vi "Obtain ACQ Data Queue.vi"(8 "error in (no error)":errorcluster) -> (0 "error out":errorcluster, 3 "ACQ Data Queue out":refnum<queue>)   [LabVIEW 2014, in "WINFAS 2 Data Queue.lvlib"]
uses:
  WINFAS 2 Data Queue.lvlib
  Acquisition Data 1 Sample Cluster.ctl
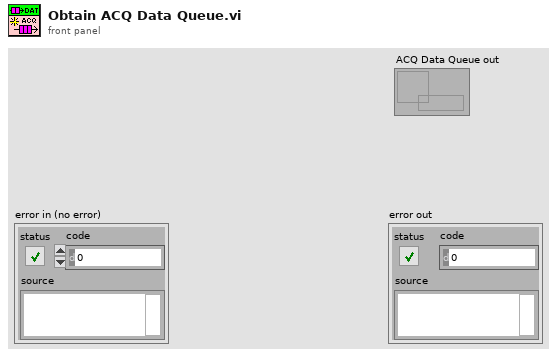
[diagram p1: front panel]
types:
  T1 = typedef "WINFAS 2 Data Queue.lvlib/Acquisition Data 1 Sample Cluster.ctl" = cluster{"TDX":sgl[], "Encoder":sgl}
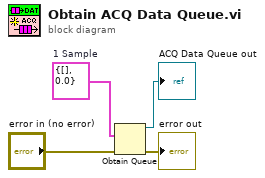
[diagram p0: block diagram]
diagram:
  w2 = T1 {"TDX"=[], "Encoder"=0.0}  # 1 Sample
  n1 = Obtain Queue(element data type=w2, error in (no error)="error in (no error)") -> (queue out=→"ACQ Data Queue out":refnum<queue>, error out=→"error out":errorcluster)  [unwired: 3 in, 1 out]
